vi "displayImage.vi"() -> ()   [LabVIEW 2016]
panel:
  out "Object Image":i32[][](graph)
  out "On Sensor Image":i32[][](graph) caption="Object Image"
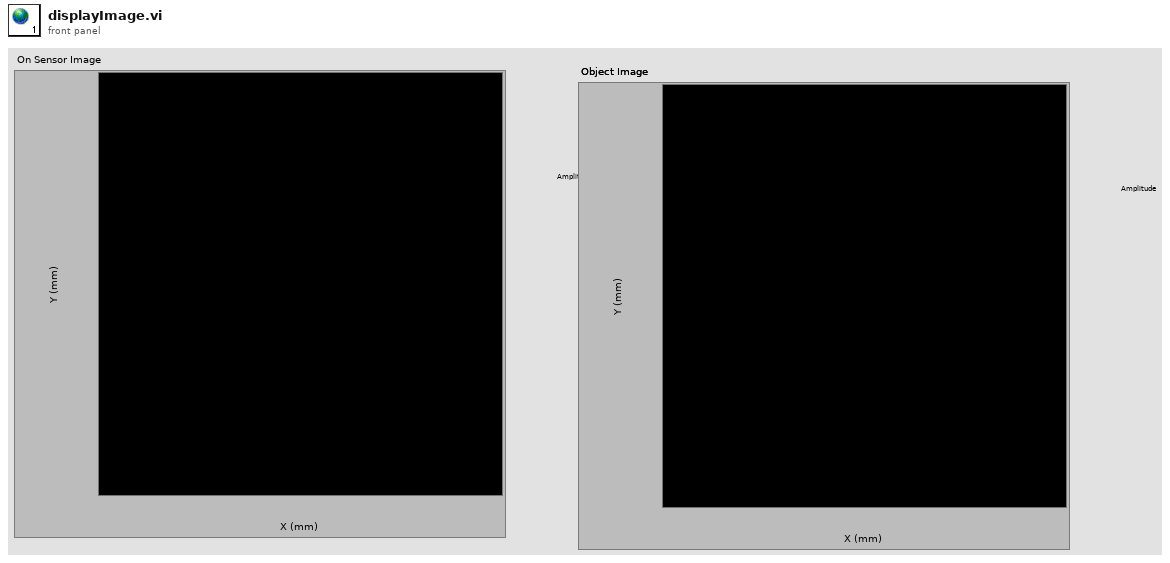
[diagram p1: front panel]
diagram:
